vi "set_from_SpaceVectors.vi"(8 "error in (no error)":errorcluster, 10 "voxels":refnum<class "SpaceVector.lvclass">[](array[class]), 11 "TrajectoryDL091126GenericVoxel in":refnum<class "TrajectoryDL091126GenericVoxel.lvclass">) -> (0 "error out":errorcluster, 3 "TrajectoryDL091126GenericVoxel out":refnum<class "TrajectoryDL091126GenericVoxel.lvclass">)   [LabVIEW 2010, in "TrajectoryDL091126GenericVoxel.lvclass"]
uses:
  TrajectoryDL091126GenericVoxel.lvclass
  common/classes/SpaceVector/SpaceVector/SpaceVector.lvclass
  common/enumerations/functional_global_action_enum.ctl
  common/enumerations/x_y_z_enumeration.ctl
  common/classes/ErrorController/ErrorController/class_data.vi
  common/classes/ErrorController/ErrorController/ErrorController.lvclass
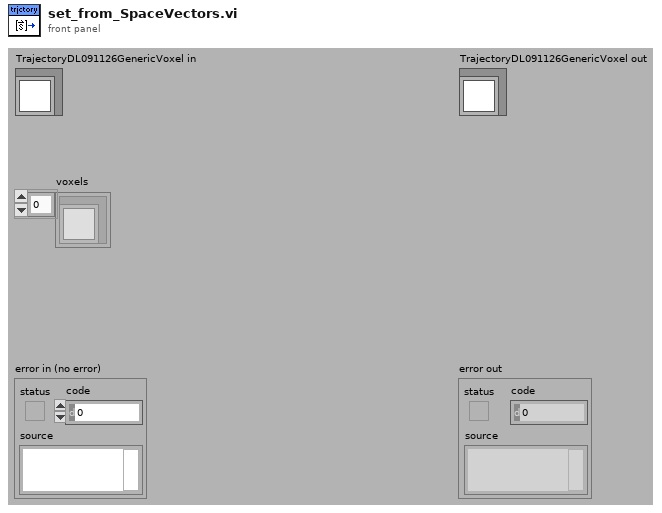
[diagram p1: front panel]
types:
  T1 = typedef "x_y_z_enumeration.ctl" = enum16{"x", "y", "z"}
  T2 = typedef "functional_global_action_enum.ctl" = enum16{"get", "set", "reset"}
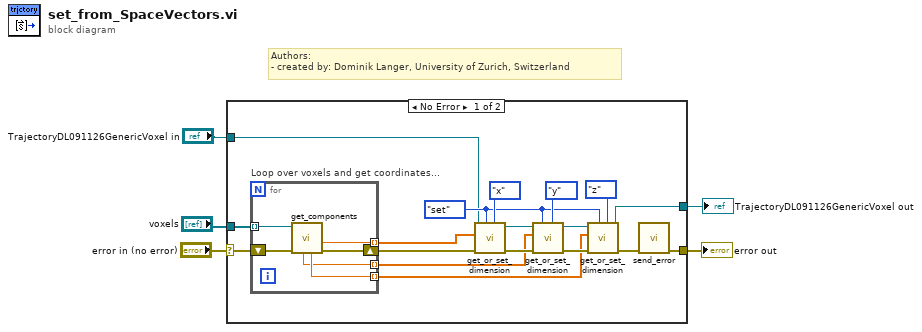
[diagram p0: block diagram]
diagram:
  # "Authors: \n- created by: Dominik Langer, University of Zurich, Switzerland"
  n1 = case shown="No Error" "error in (no error)" {
    selector: "error in (no error)" -> [w15 w31]
    tunnel: [w6 w31] -> w4
    tunnel: [w8 w30] -> w2
    tunnel: "TrajectoryDL091126GenericVoxel in" -> [w9 w30]
    tunnel: "voxels" -> [w13 _]
    frame No Error {
      w16 = functional_global_action_enum."set" ("action")
      n2 = for "Loop over voxels and get coordinates..." {
        tunnel: w13 -> [w27] mode=indexing
        shift-right: [w28] -> w14
        shift-left: w15 -> [w29]
        tunnel: [w26] -> w11 mode=indexing
        tunnel: [w25] -> w12 mode=indexing
        tunnel: [w24] -> w10 mode=indexing
        n3 = call "get_components.vi"("error in (no error)"=w29, "SpaceVector in"=w27) -> ("error out"=w28:errorcluster, "x"=w26:dbl[unit], "z"=w25:dbl[unit], "y"=w24:dbl[unit])  [unwired: 4 in, 2 out]
      }
      n4 = call-dynamic "get_or_set_dimension.vi"("dimension"=x_y_z_enumeration."x", "action"=w16, "error in (no error)"=w14, "pixel values in (single dimension)"=w11, "GenericTrajectory in"=w9) -> ("error out"=w23:errorcluster, "GenericTrajectory out"=w21:refnum<class "TrajectoryDL091126GenericVoxel.lvclass">)  [unwired: 4 in, 1 out]
      n5 = call-dynamic "get_or_set_dimension.vi"("dimension"=x_y_z_enumeration."y", "action"=w16, "error in (no error)"=w23, "pixel values in (single dimension)"=w10, "GenericTrajectory in"=w21) -> ("error out"=w22:errorcluster, "GenericTrajectory out"=w20:refnum<class "TrajectoryDL091126GenericVoxel.lvclass">)  [unwired: 4 in, 1 out]
      n6 = call-dynamic "get_or_set_dimension.vi"("dimension"=x_y_z_enumeration."z", "action"=w16, "error in (no error)"=w22, "pixel values in (single dimension)"=w12, "GenericTrajectory in"=w20) -> ("error out"=w7:errorcluster, "GenericTrajectory out"=w8:refnum<class "TrajectoryDL091126GenericVoxel.lvclass">)  [unwired: 4 in, 1 out]
      n7 = call "send_error.vi"("error in (no error)"=w7) -> ("error out"=w6:errorcluster)  [unwired: 10 in]
    }
    frame Error {
    }
  }
  "error out" <- w4
  "TrajectoryDL091126GenericVoxel out" <- w2
